vi "WebDAV FGV.vi"(7 "WebDAV States":T3=enum."Create Dir", 8 "error in (no error)":errorcluster, 9 "local file path":path, 10 "host uri prefix":string="http://192.168.1.10/files", 11 "relative uri":string="/C/TTV Test Patterns/") -> (0 "error out":errorcluster={"status"=TRUE, "code"=-1967362020, "source"="NI_WebDAV.lvlib:Create Directory.vi:5520001<APPEND>\n\n<b>Complete call chain:</b>\r\n     NI_WebDAV.lvlib:Create Directory.vi:5520001\r\n     Cobra Single Head GUI.lvlib:WebDAV FGV.vi"}, 2 "file list":T2[](array[typedef]), 3 "session handle out":T1)   [LabVIEW 2019, in "GUI.lvlib"]
uses:
  GUI.lvlib
  Controls/WebDAV states.ctl
  <vilib>/WebDAVClient/Advanced/FileInfo.ctl
  <vilib>/WebDAVClient/Advanced/SessionHandle.ctl
  <vilib>/WebDAVClient/Advanced/Get File.vi
  <vilib>/WebDAVClient/Advanced/Put File.vi
  <vilib>/WebDAVClient/NI_WebDAV.lvlib
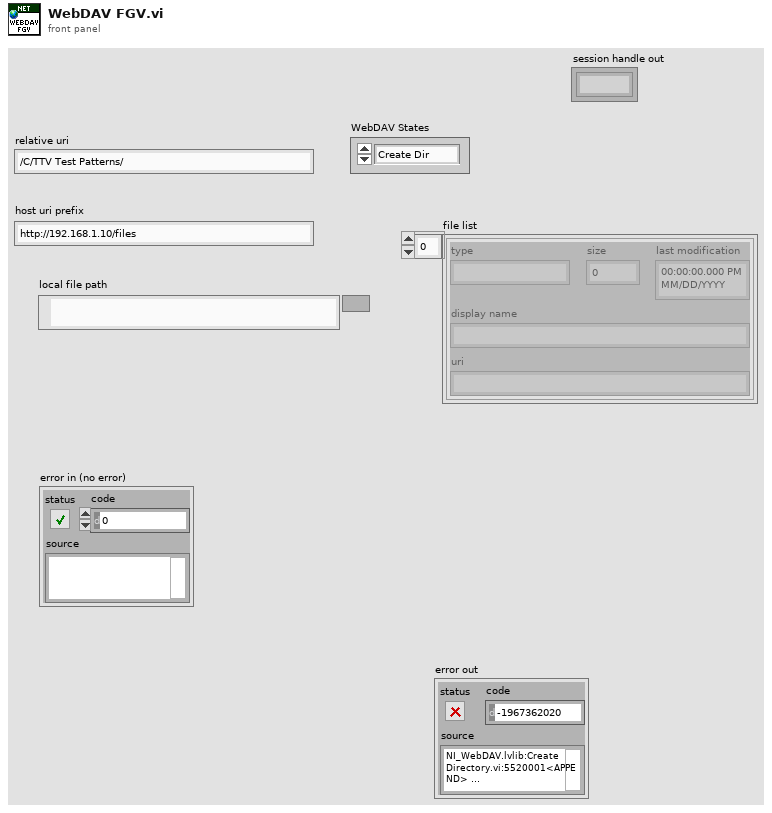
[diagram p1: front panel]
types:
  T1 = typedef "NI_WebDAV.lvlib/SessionHandle.ctl" = refnum<k1>
  T2 = typedef "NI_WebDAV.lvlib/FileInfo.ctl" = cluster{"type":string, "size":u64, "last modification":timestamp, "display name":string, "uri":string}
  T3 = typedef "GUI.lvlib/WebDAV states.ctl" = enum16{"Open Sess", "Refresh Dir", "Create Dir", "Upload", "Download", "Delete", "Close Sess"}
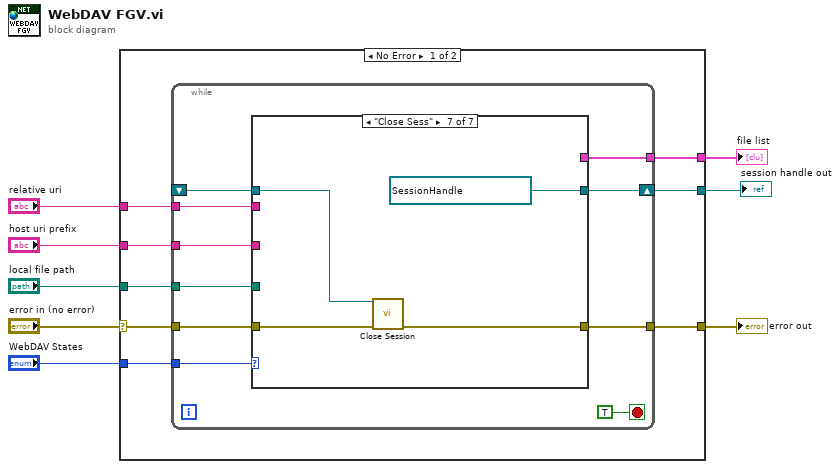
[diagram p0: block diagram]
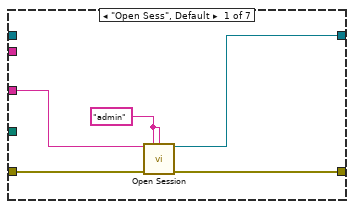
[diagram p2: hidden frame]
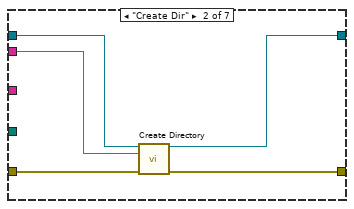
[diagram p3: hidden frame]
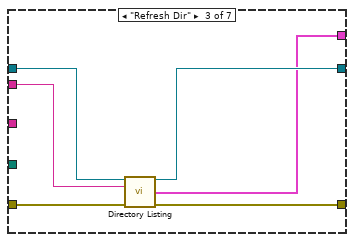
[diagram p4: hidden frame]
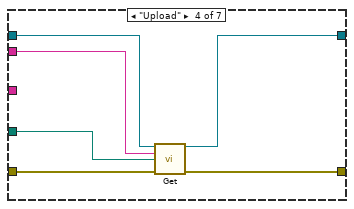
[diagram p5: hidden frame]
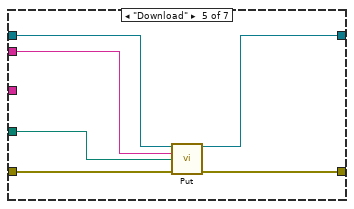
[diagram p6: hidden frame]
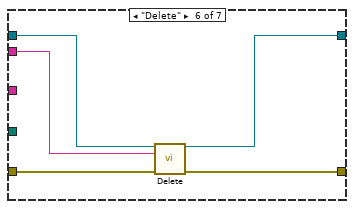
[diagram p7: hidden frame]
diagram:
  n1 = case shown="No Error" "error in (no error)" {
    selector: "error in (no error)" -> [w11 w64]
    tunnel: [w16 w64] -> w8
    tunnel: "WebDAV States" -> [w15 _]
    tunnel: "host uri prefix" -> [w14 _]
    tunnel: "relative uri" -> [w13 _]
    tunnel: "local file path" -> [w10 _]
    tunnel: [w12 _] -> w3
    tunnel: [w9 _] -> w1
    frame No Error {
      n2 = while {
        tunnel: w15 -> [w24]
        tunnel: w14 -> [w23]
        tunnel: w13 -> [w21]
        tunnel: w11 -> [w26]
        tunnel: [w25] -> w16
        shift-right: [w22] -> w9
        shift-left: _ -> [w18]
        tunnel: [w20] -> w12
        tunnel: w10 -> [w17]
        stop <- TRUE stop-if-true
        n3 = case shown="\"Close Sess\"" w24 {
          tunnel: w26 -> [w31 w36 w42 w48 w54 w59 w62]
          tunnel: [w27 w33 w38 w46 w50 w56 w63] -> w22
          tunnel: w18 -> [_ w34 w39 w45 w52 w57 w60]
          tunnel: [w28 w35 w41 w47 w53 w58 w61] -> w25
          tunnel: w23 -> [w29 _ _ _ _ _ _]
          tunnel: w21 -> [_ w32 w40 w44 w51 w55 _]
          tunnel: [_ _ w37 _ _ _ _] -> w20
          tunnel: w17 -> [_ _ _ w43 w49 _ _]
          frame "Open Sess", Default {
            w30 = "admin" ("username")
            n4 = call <vilib>:"Open Session.vi"("host uri prefix"=w29, "username"=w30, "password"=w30, "error in (no error)"=w31) -> ("session handle out"=w27:T1, "error out"=w28:errorcluster)  [unwired: 10 in]
          }
          frame "Create Dir" {
            n5 = call <vilib>:"Create Directory.vi"("session handle"=w34, "relative uri"=w32, "error in (no error)"=w36) -> ("session handle out"=w33:T1, "error out"=w35:errorcluster)  [unwired: 11 in]
          }
          frame "Refresh Dir" {
            n6 = call <vilib>:"Directory Listing.vi"("session handle"=w39, "relative uri"=w40, "error in (no error)"=w42) -> ("session handle out"=w38:T1, "file list"=w37:T2[], "error out"=w41:errorcluster)  [unwired: 9 in, 1 out]
          }
          frame "Upload" {
            n7 = call-poly <vilib>:"Get.vi"("session handle"=w45, "relative uri"=w44, "local file path"=w43, "error in (no error)"=w48) -> ("session handle out"=w46:T1, "error out"=w47:errorcluster)  [unwired: 9 in, 1 out]
          }
          frame "Download" {
            n8 = call-poly <vilib>:"Put.vi"("session handle"=w52, "relative uri"=w51, "local file path"=w49, "error in (no error)"=w54) -> ("session handle out"=w50:T1, "error out"=w53:errorcluster)  [unwired: 9 in, 1 out]
          }
          frame "Delete" {
            n9 = call <vilib>:"Delete.vi"("session handle"=w57, "relative uri"=w55, "error in (no error)"=w59) -> ("session handle out"=w56:T1, "error out"=w58:errorcluster)  [unwired: 11 in]
          }
          frame "Close Sess" {
            w63 = T1 refnum items=["Session NI_WebDAV"] ("session handle out")
            n10 = call <vilib>:"Close Session.vi"("session handle"=w60, "error in (no error)"=w62) -> ("error out"=w61:errorcluster)  [unwired: 13 in]
          }
        }
      }
    }
    frame Error {
    }
  }
  "error out" <- w8
  "file list" <- w3
  "session handle out" <- w1
